vi "AcqVideoOptCodes.vi"(8 "error in (no error)":errorcluster, 11 "CameraTestingProxyAPI in":refnum<class "CameraTestingProxyAPI.lvclass">) -> (0 "error out":errorcluster, 2 "VideoOptionsInfo":T1, 3 "CameraTestingProxyAPI out":refnum<class "CameraTestingProxyAPI.lvclass">)   [LabVIEW 2020, in "CameraTestingProxy.lvlib" / "CameraTestingProxyAPI.lvclass"]
uses:
  CameraTestingProxyAPI.lvclass
  CameraTestingApp/ICameraTesting/ICameraTesting/TypeDef/VideoOptionsInfo.ctl
  CameraTestingProxyAPI.lvclass/CameraTestingProxyAPI.ctl
  79a1970e-1e8b-4eff-b328-15511f37bcfa.vi
  CameraTestingApp/ICameraTesting/ICameraTesting/ICameraTesting.lvclass
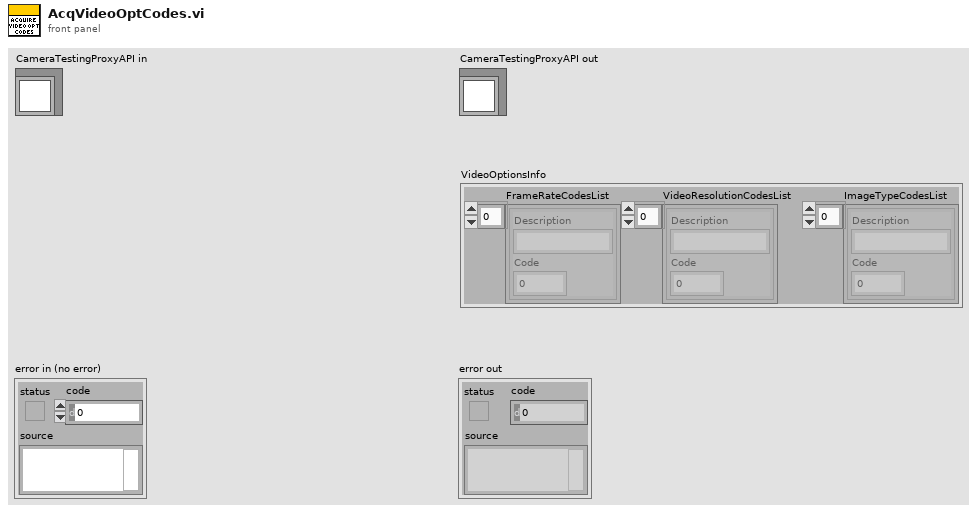
[diagram p1: front panel]
types:
  T1 = typedef "ICameraTesting.lvlib/ICameraTesting.lvclass/VideoOptionsInfo.ctl" = cluster{"FrameRateCodesList":cluster{"Description":string, "Code":u8}[], "VideoResolutionCodesList":cluster{"Description":string, "Code":u8}[], "ImageTypeCodesList":cluster{"Description":string, "Code":u8}[]}
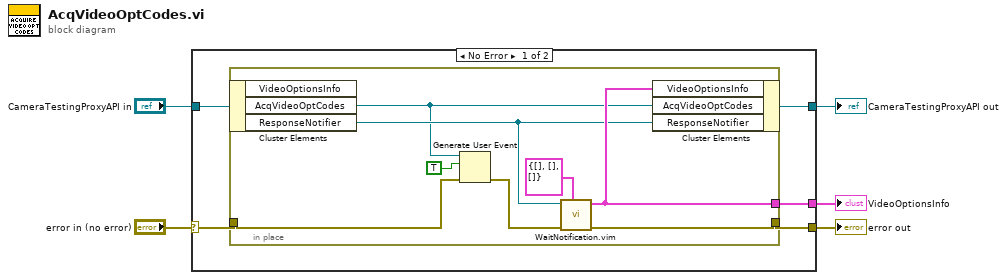
[diagram p0: block diagram]
diagram:
  n1 = case shown="No Error" "error in (no error)" {
    selector: "error in (no error)" -> [w10 w20]
    tunnel: [w8 w20] -> w2
    tunnel: [w6 w19] -> w5
    tunnel: "CameraTestingProxyAPI in" -> [w7 w19]
    tunnel: [w9 _] -> w1
    frame No Error {
      n2 = in-place {
        in-place-border: w10 -> [w18]
        in-place-border: [w13] -> w9
        in-place-border: [w15] -> w8
        n3 = in-place-cluster #1(w7) -> ("AcqVideoOptCodes"=w11:refnum<user-event>, "ResponseNotifier"=w12:refnum<notifier>)  [unwired: 1 out]
        n4 = Generate User Event(user event=w11, event data cluster=TRUE ("event data"), error in=w18) -> (error out=w16:errorcluster)  [unwired: 1 in, 1 out]
        n5 = call "WaitNotification.vim"("Type"=T1 {"FrameRateCodesList"=[], "VideoResolutionCodesList"=[], "ImageTypeCodesList"=[]} ("VideoOptionsInfo"), "error in (no error)"=w16, "ResponseNotifier"=w12) -> ("error out"=w15:errorcluster, "Data"=w13:T1)  [unwired: 7 in]
        n6 = in-place-cluster #1("VideoOptionsInfo"=w13, "AcqVideoOptCodes"=w11, "ResponseNotifier"=w12) -> (w6:refnum<class "CameraTestingProxyAPI.lvclass">)
      }
    }
    frame Error {
    }
  }
  "error out" <- w2
  "CameraTestingProxyAPI out" <- w5
  "VideoOptionsInfo" <- w1
